vi "Dictionary.vi"(8 "error in":errorcluster, 9 "Value":variant, 10 "Key":string, 11 "Command":string) -> (0 "error out":errorcluster, 3 "Value Out":variant)   [LabVIEW 2015]
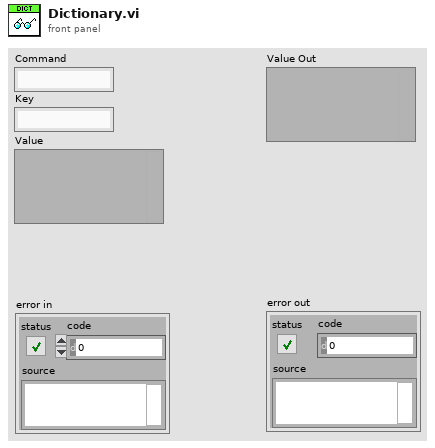
[diagram p1: front panel]
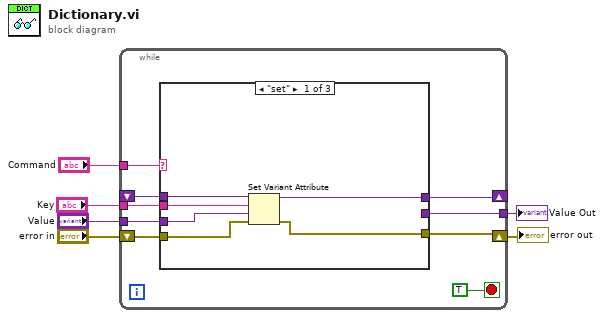
[diagram p0: block diagram]
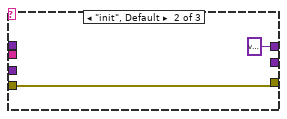
[diagram p2: hidden frame]
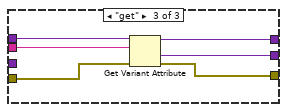
[diagram p3: hidden frame]
diagram:
  n1 = while {
    tunnel: "Command" -> [w14]
    shift-right: [w12] -> _
    shift-left: _ -> [w13]
    tunnel: "Key" -> [w11]
    tunnel: "Value" -> [w10]
    tunnel: [w7] -> w2
    shift-right: [w8] -> w1
    shift-left: "error in" -> [w9]
    stop <- TRUE stop-if-true
    n2 = case shown="\"set\"" w14 {
      tunnel: w13 -> [w21 _ w29]
      tunnel: [w20 variant ("Variant") w28] -> w12
      tunnel: w11 -> [w19 _ w27]
      tunnel: w10 -> [w18 _ _]
      tunnel: w9 -> [w17 w22 w26]
      tunnel: [w16 w22 w25] -> w8
      tunnel: [_ _ w24] -> w7
      frame "set" {
        n3 = Set Variant Attribute(Variant=w21, name=w19, value=w18, error in=w17) -> (Variant out=w20:variant, error out=w16:errorcluster)  [unwired: 1 out]
      }
      frame "init", Default {
      }
      frame "get" {
        n4 = Get Variant Attribute(Variant=w29, name=w27, error in=w26) -> (duplicate Variant=w28:variant, value=w24:variant, error out=w25:errorcluster)  [unwired: 1 in, 1 out]
      }
    }
  }
  "Value Out" <- w2
  "error out" <- w1
